vi "displayDialog.vi"(11 "String In":string) -> (3 "String Out":string)   [LabVIEW 2019]
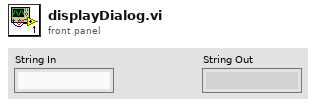
[diagram p1: front panel]
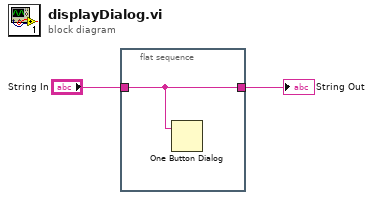
[diagram p0: block diagram]
diagram:
  n1 = flat-sequence {
    tunnel: "String In" -> [w3]
    tunnel: [w3] -> w1
    frame #0 {
      n2 = One Button Dialog(message=w3) -> ()  [unwired: 1 in, 1 out]
    }
  }
  "String Out" <- w1
